vi "SerialPort_Read.vi"(2 "error in":errorcluster, 3 "COM Port":refnum<visa-resource-name>) -> (0 "error out":errorcluster, 1 "read buffer":string)   [LabVIEW 2015]
uses:
  <vilib>/Instr/_visa.llb/VISA Configure Serial Port (Instr).vi
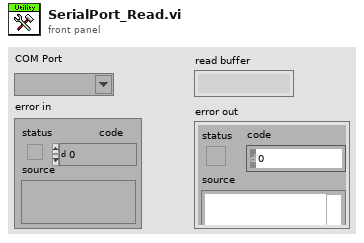
[diagram p1: front panel]
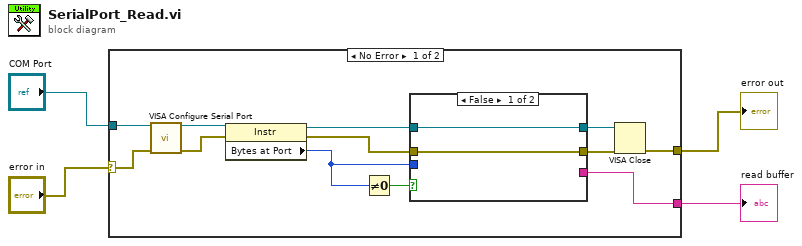
[diagram p0: block diagram]
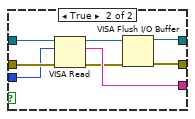
[diagram p2: hidden frame]
diagram:
  n1 = case shown="No Error" "error in" {
    selector: "error in" -> [w8 _]
    tunnel: "COM Port" -> [w7 _]
    tunnel: [w6 _] -> w2
    tunnel: [w5 _] -> w1
    frame No Error {
      n2 = call-poly "VISA Configure Serial Port"("VISA resource name"=w7, "error in (no error)"=w8) -> ("VISA resource name out"=w16:refnum<visa-resource-name>, "error out"=w13:errorcluster)  [unwired: 12 in]
      n3 = property class="Instr"(reference=w16, error in=w13) -> (reference out=w14:refnum<visa-resource-name>, error out=w15:errorcluster, "Bytes at Port"=w11:u32)
      n4 = Not Equal To 0?(x=w11) -> (x != 0?=w12:bool)
      n5 = case shown="False" w12 {
        tunnel: w15 -> [w17 w26]
        tunnel: w14 -> [w18 w25]
        tunnel: w11 -> [_ w24]
        tunnel: [w18 w20] -> w10
        tunnel: [w17 w22] -> w9
        tunnel: [_ w23] -> w5
        frame False {
        }
        frame True {
          n6 = VISA Read(VISA resource name=w25, byte count=w24, error in (no error)=w26) -> (VISA resource name out=w21:refnum<visa-resource-name>, read buffer=w23:string, error out=w19:errorcluster)  [unwired: 1 out]
          n7 = VISA Flush I/O Buffer(VISA resource name=w21, error in (no error)=w19) -> (VISA resource name out=w20:refnum<visa-resource-name>, error out=w22:errorcluster)  [unwired: 1 in]
        }
      }
      n8 = VISA Close(VISA resource name=w10, error in (no error)=w9) -> (error out=w6:errorcluster)
    }
    frame Error {
    }
  }
  "error out" <- w2
  "read buffer" <- w1
